vi "iTC_Readout (2).vi"() -> ()   [LabVIEW 2009]
panel:
  out "millisecond timer value":u32
  out "CCS Resistance":dynamicdata(graph)
  out "CCS Temperature":dbl(slide) scale=0.0..100.0
  in  "Samples Per Second 6":dbl=15.0
  out "CCS Temperature":string
  out "CCS Resistance":dbl(knob) scale=0.0..500.0
  out "CCS Resistance":string
  out "CCS Temperature":dynamicdata(graph)
  in  "Samples Per Second 5":dbl=15.0
  out "Allen Bradley Temperature":dbl(slide) scale=0.0..500.0
  out "Allen Bradley Temperature":string
  out "Allen Bradley Temperature":dynamicdata(graph)
  in  "Samples Per Second 4":dbl=15.0
  out "Allen Bradley Resistance":dbl(knob) scale=0.3..300.0
  out "Allen Bradley Resistance":string
  out "Allen Bradley Resistance":dynamicdata(graph)
  in  "Samples Per Second 3":dbl=15.0
  in  "Samples Per Second 2":dbl=15.0
  in  "Samples Per Second":dbl=15.0
  in  "stop 2":bool
  out "Heartbeat":bool
  out "Cernox Temp":string
  out "Cernox Temperature":dynamicdata(graph)
  out "Cernox Temp":dbl(slide) scale=0.0..320.0
  out "Cernox Resistance":dynamicdata(graph)
  out "Cernox Resistance":dbl(knob) scale=0.0..300.0
  out "Cernox Resistance":string
  in  "stop":bool
  out "Measurement":bool caption="Taken"
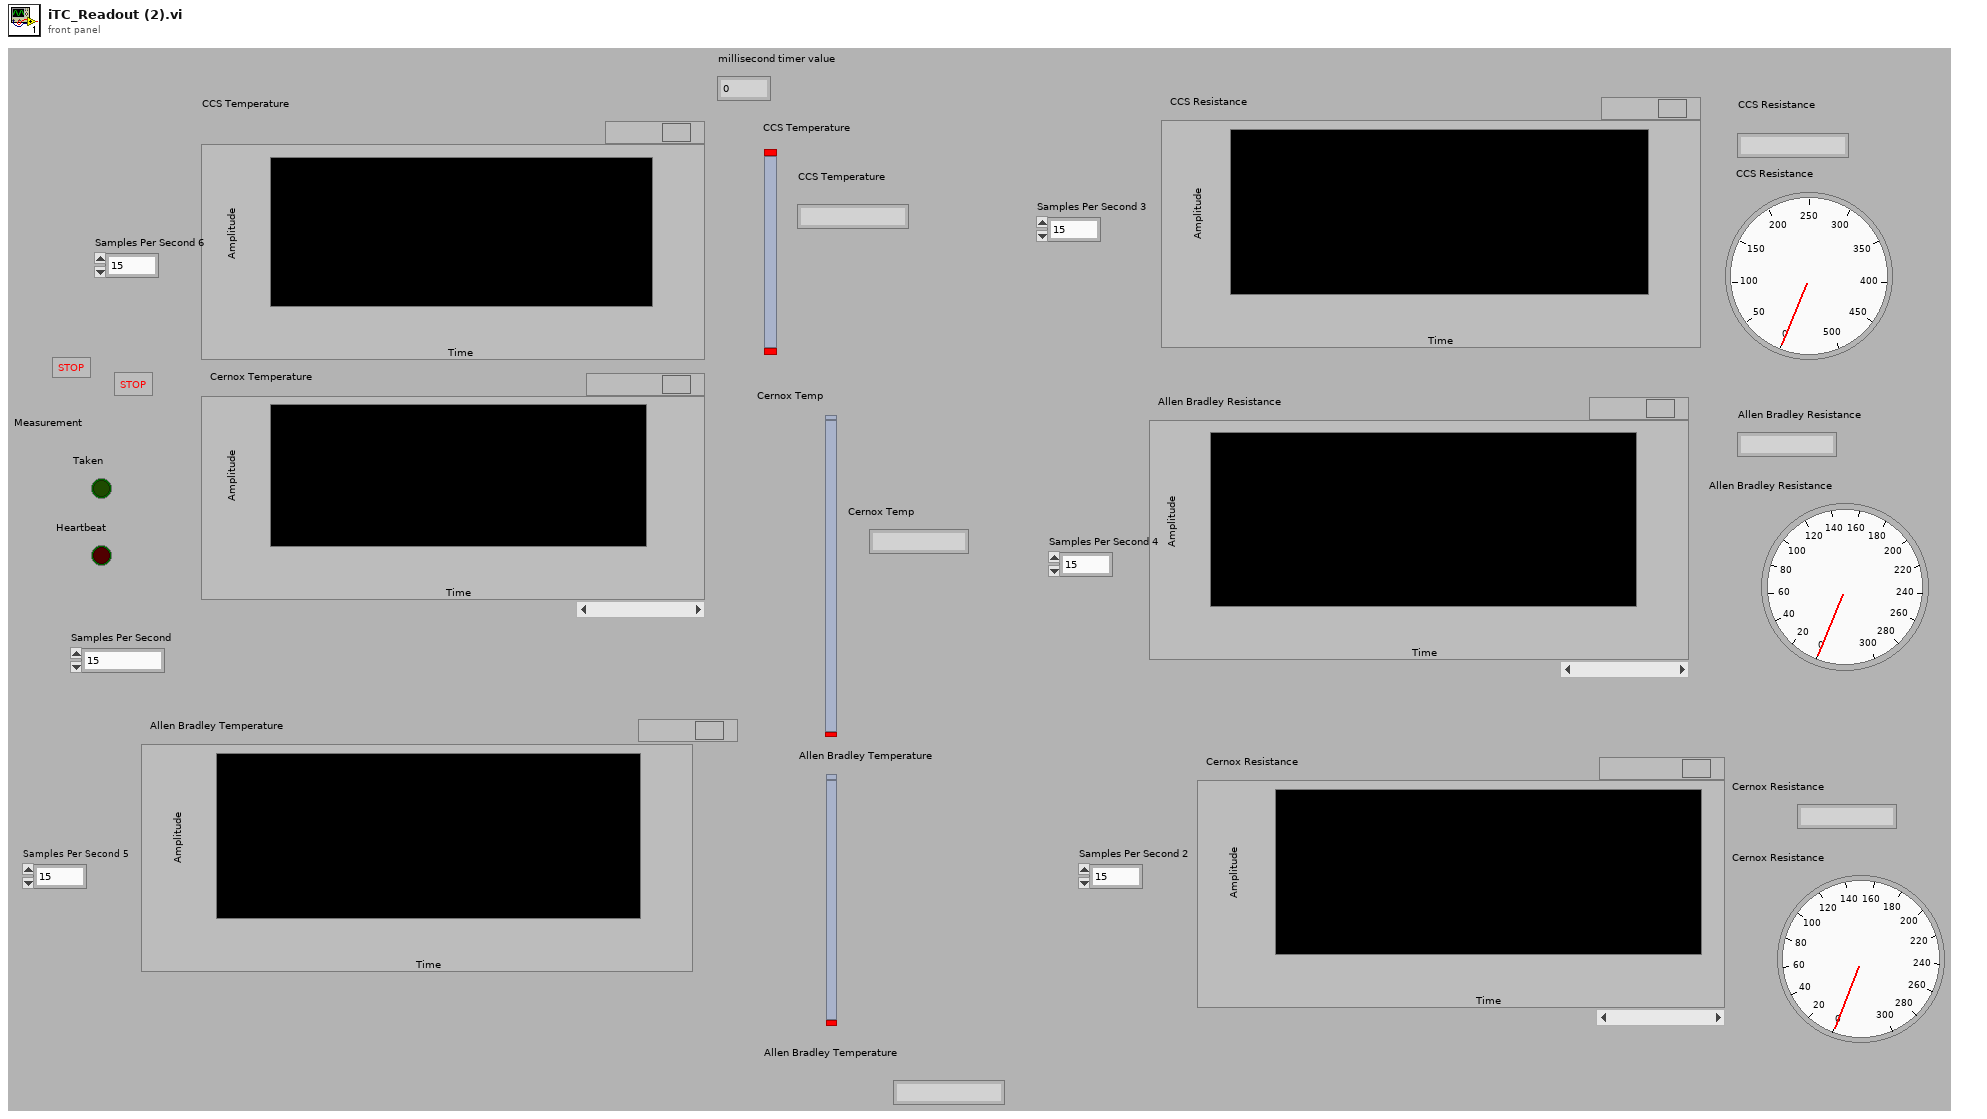
[diagram p1: front panel]
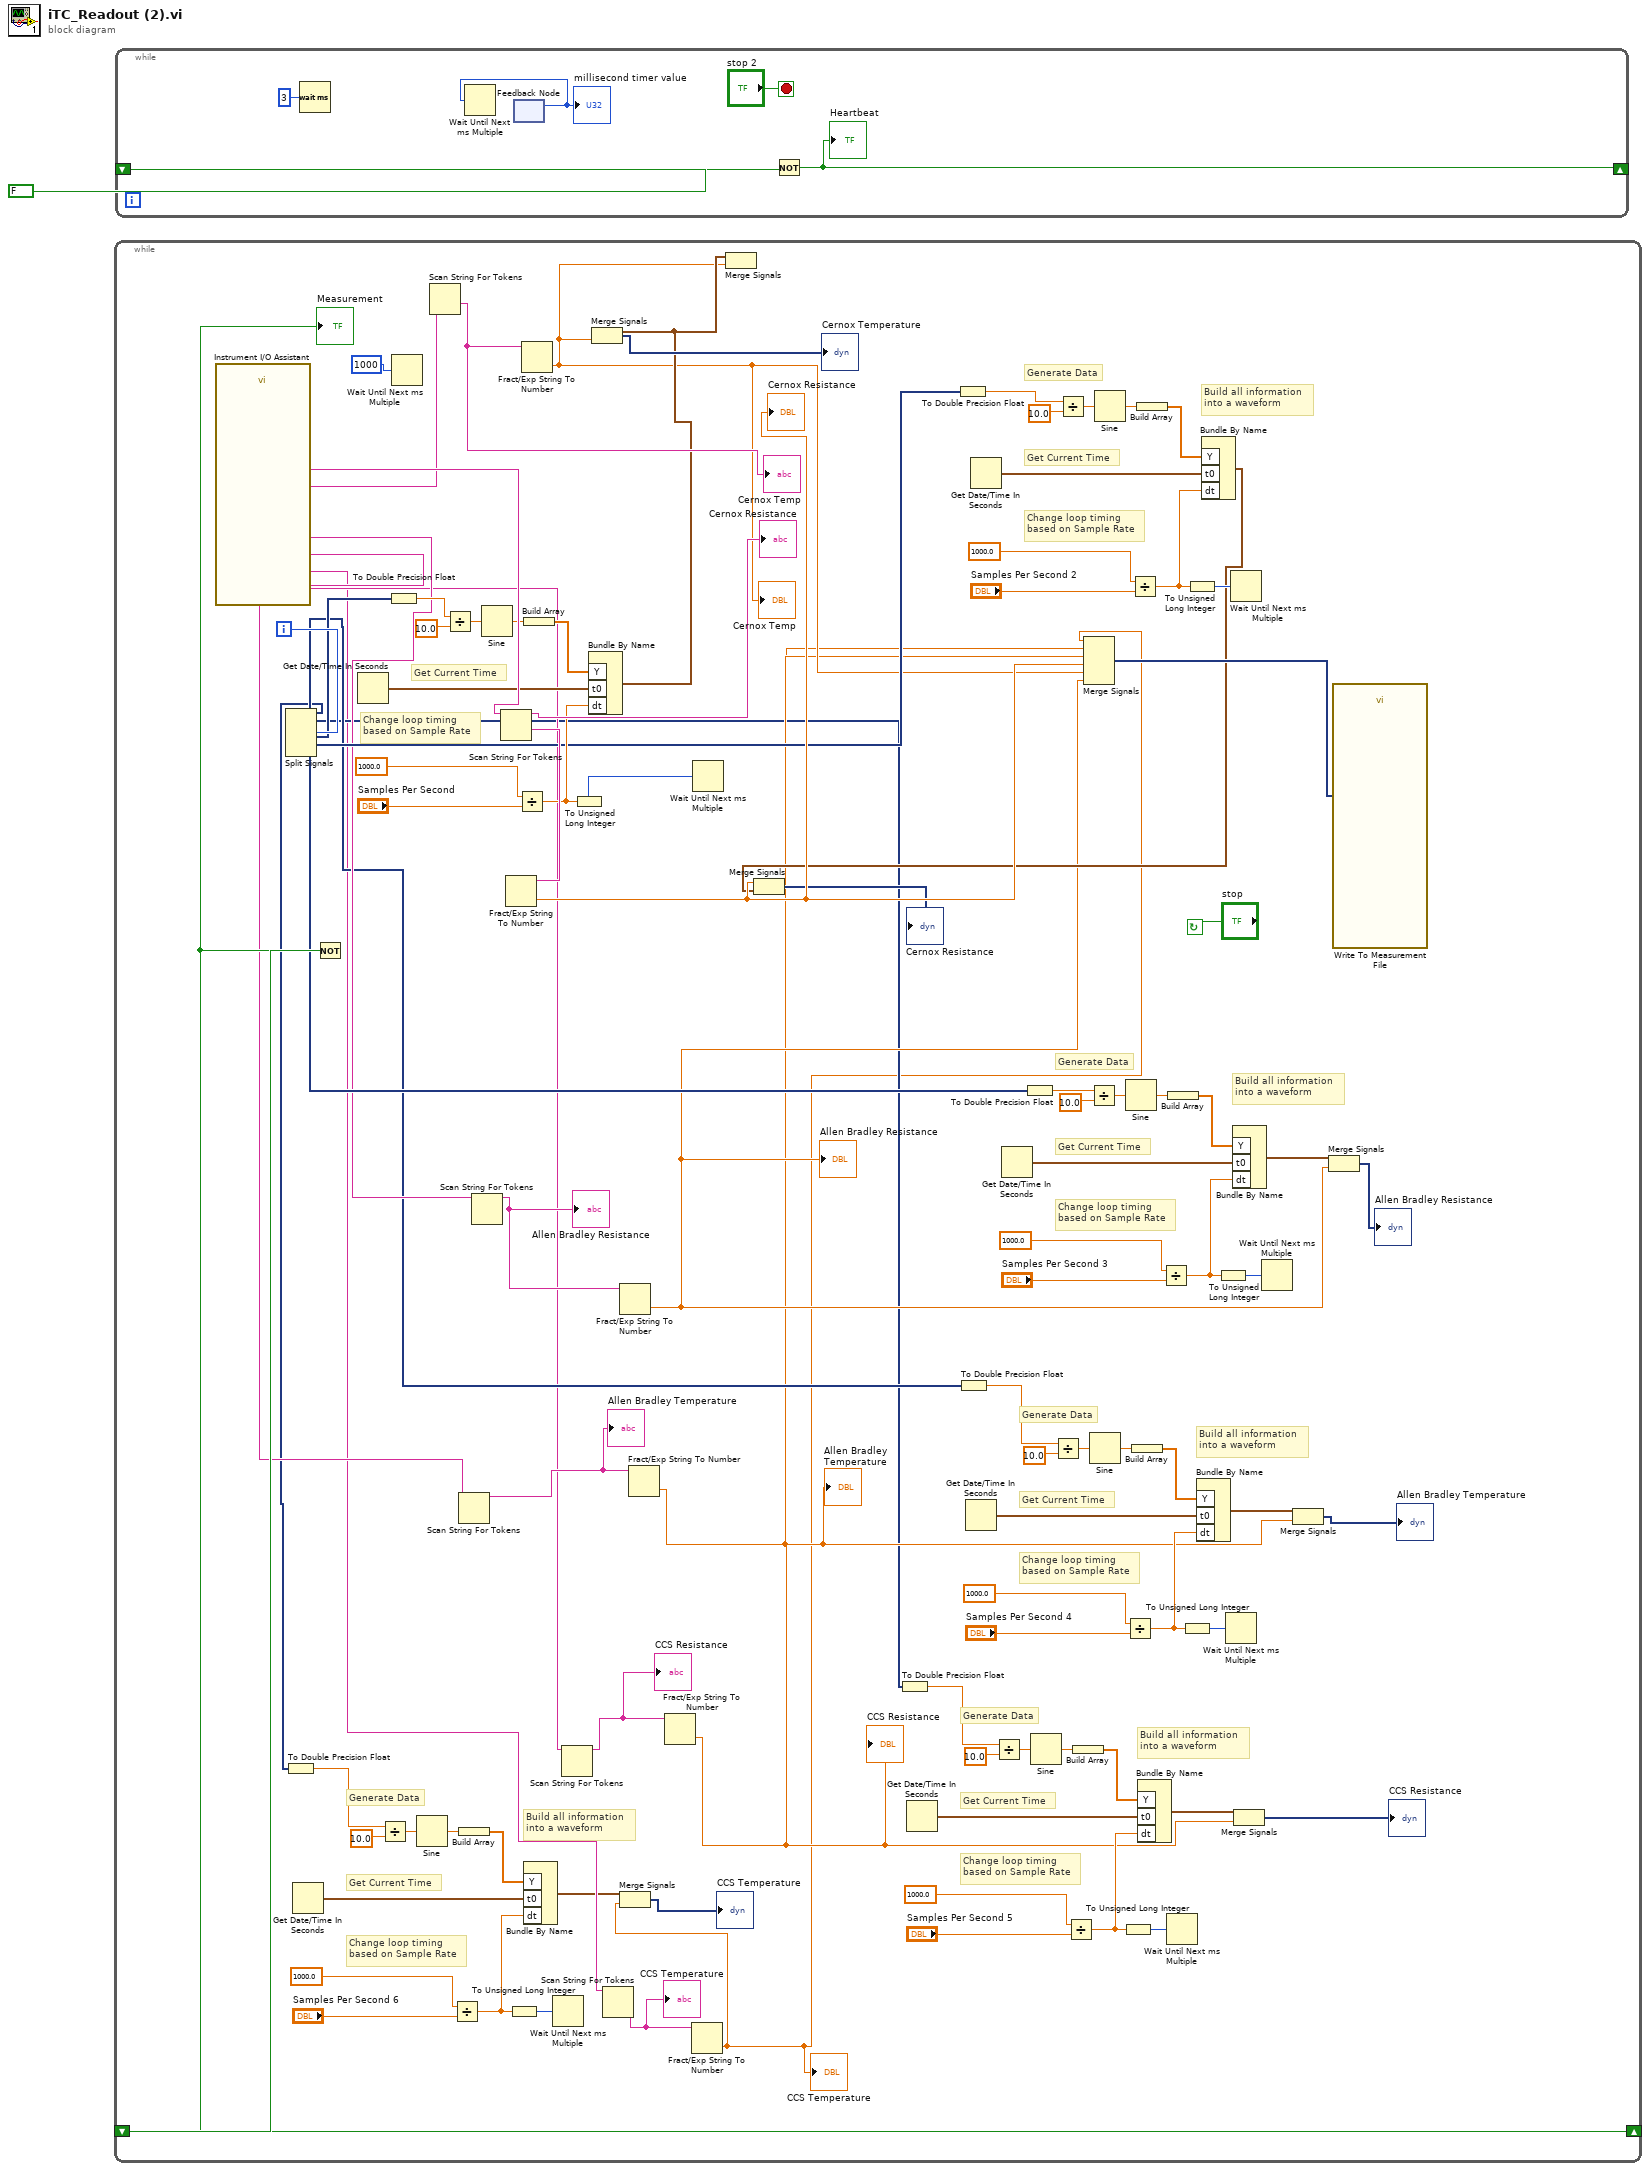
[diagram p0: block diagram]
diagram:
  n1 = while {
    shift-right: [w103] -> _
    shift-left: _ -> [w104]
    i -> [w70]
    stop <- "stop" continue-if-true
    # "Build all information\ninto a waveform"
    # "Change loop timing\nbased on Sample Rate"
    # "Get Current Time"
    # "Generate Data"
    # "Build all information\ninto a waveform"
    # "Change loop timing\nbased on Sample Rate"
    # "Get Current Time"
    # "Generate Data"
    # "Build all information\ninto a waveform"
    # "Change loop timing\nbased on Sample Rate"
    # "Get Current Time"
    # "Generate Data"
    # "Build all information\ninto a waveform"
    # "Change loop timing\nbased on Sample Rate"
    # "Get Current Time"
    # "Generate Data"
    # "Build all information\ninto a waveform"
    # "Change loop timing\nbased on Sample Rate"
    # "Get Current Time"
    # "Generate Data"
    # "Change loop timing\nbased on Sample Rate"
    # "Get Current Time"
    n2 = call "Instrument I/O Assistant"() -> ("token"=w22:string, "CCS Temperature"=w18:string, "Allen Bradley Temperature"=w37:string, "Allen Bradley Resistance"=w53:string, "Cernox Temp"=w99:string, "Cernox Resistance"=w101:string)  [unwired: 21 in, 1 out]
    n3 = Split Signals(w70) -> (w4:dynamicdata, w20:dynamicdata, w35:dynamicdata, w69:dynamicdata, w68:dynamicdata, w55:dynamicdata)  [unwired: 6 in]
    n4 = To Double Precision Float(number=w4) -> (double precision float=w10:dbl)
    n5 = Get Date/Time In Seconds() -> (seconds since 1Jan1904=w15:timestamp)
    n6 = Not(x=w104) -> (.not. x?=w103:bool)
    "Measurement" <- w103
    n7 = Get Date/Time In Seconds() -> (seconds since 1Jan1904=w85:timestamp)
    n8 = Divide(x=w10, y=10.0) -> (x/y=w7:dbl)
    n9 = To Double Precision Float(number=w69) -> (double precision float=w90:dbl)
    n10 = Wait Until Next ms Multiple(millisecond multiple=u32 1000) -> ()  [unwired: 1 out]
    n11 = Sine(x=w7) -> (sin(x)=w13:dbl)
    n12 = Scan String For Tokens(9:w99) -> (1:w97:string)  [unwired: 5 in, 3 out]
    "Cernox Temp" <- w97
    n13 = Divide(x=w90, y=10.0) -> (x/y=w93:dbl)
    n14 = Divide(x=1000.0, y="Samples Per Second 6") -> (x/y=w16:dbl)
    n15 = Scan String For Tokens(9:w37) -> (3:w36:string)  [unwired: 5 in, 3 out]
    "Allen Bradley Temperature" <- w36
    n16 = Build Array(w13) -> (w14:dbl[])
    n17 = Scan String For Tokens(9:w53) -> (3:w51:string)  [unwired: 5 in, 3 out]
    "Allen Bradley Resistance" <- w51
    n18 = Sine(x=w93) -> (sin(x)=w87:dbl)
    n19 = Scan String For Tokens(9:w101) -> (1:w100:string, 3:→"Cernox Resistance":string)  [unwired: 5 in, 2 out]
    n20 = Fract/Exp String To Number(string=w100) -> (number=w73:dbl)  [unwired: 3 in, 1 out]
    "Cernox Resistance" <- w73
    n21 = To Unsigned Long Integer(number=w16) -> (unsigned 32bit integer=w9:u32)
    n22 = Divide(x=1000.0, y="Samples Per Second") -> (x/y=w84:dbl)
    n23 = Fract/Exp String To Number(string=w97) -> (number=w66:dbl)  [unwired: 3 in, 1 out]
    "Cernox Temp" <- w66
    n24 = Build Array(w87) -> (w86:dbl[])
    n25 = Bundle By Name("Y"=w14, "t0"=w15, "dt"=w16) -> (w6:waveform(dbl))  [unwired: 1 in]
    n26 = Wait Until Next ms Multiple(millisecond multiple=w9) -> ()  [unwired: 1 out]
    n27 = Scan String For Tokens(9:w22) -> (3:w21:string)  [unwired: 5 in, 3 out]
    "CCS Resistance" <- w21
    n28 = To Unsigned Long Integer(number=w84) -> (unsigned 32bit integer=w91:u32)
    n29 = Bundle By Name("Y"=w86, "t0"=w85, "dt"=w84) -> (w67:waveform(dbl))  [unwired: 1 in]
    n30 = Merge Signals(w67, w66) -> (→"Cernox Temperature":dynamicdata)
    n31 = Scan String For Tokens(9:w18) -> (3:w17:string)  [unwired: 5 in, 3 out]
    "CCS Temperature" <- w17
    n32 = Fract/Exp String To Number(string=w51) -> (number=w50:dbl)  [unwired: 3 in, 1 out]
    "Allen Bradley Resistance" <- w50
    n33 = Fract/Exp String To Number(string=w36) -> (number=w34:dbl)  [unwired: 3 in, 1 out]
    "Allen Bradley Temperature" <- w34
    n34 = Fract/Exp String To Number(string=w21) -> (number=w19:dbl)  [unwired: 3 in, 1 out]
    "CCS Resistance" <- w19
    n35 = Fract/Exp String To Number(string=w17) -> (number=w3:dbl)  [unwired: 3 in, 1 out]
    "CCS Temperature" <- w3
    n36 = Merge Signals(w6, w3) -> (→"CCS Temperature":dynamicdata)
    n37 = Wait Until Next ms Multiple(millisecond multiple=w91) -> ()  [unwired: 1 out]
    n38 = Merge Signals(w67, w66) -> ()  [unwired: 1 out]
    n39 = To Double Precision Float(number=w20) -> (double precision float=w27:dbl)
    n40 = Get Date/Time In Seconds() -> (seconds since 1Jan1904=w32:timestamp)
    n41 = To Double Precision Float(number=w68) -> (double precision float=w77:dbl)
    n42 = To Double Precision Float(number=w35) -> (double precision float=w43:dbl)
    n43 = Get Date/Time In Seconds() -> (seconds since 1Jan1904=w48:timestamp)
    n44 = Get Date/Time In Seconds() -> (seconds since 1Jan1904=w82:timestamp)
    n45 = Divide(x=w27, y=10.0) -> (x/y=w24:dbl)
    n46 = Get Date/Time In Seconds() -> (seconds since 1Jan1904=w64:timestamp)
    n47 = To Double Precision Float(number=w55) -> (double precision float=w59:dbl)
    n48 = Sine(x=w24) -> (sin(x)=w30:dbl)
    n49 = Divide(x=w43, y=10.0) -> (x/y=w40:dbl)
    n50 = Divide(x=w77, y=10.0) -> (x/y=w74:dbl)
    n51 = Divide(x=1000.0, y="Samples Per Second 5") -> (x/y=w33:dbl)
    n52 = Build Array(w30) -> (w31:dbl[])
    n53 = Merge Signals(w3, w19, w34, w73, w66, w50) -> (w98:dynamicdata)
    n54 = Divide(x=w59, y=10.0) -> (x/y=w56:dbl)
    n55 = Sine(x=w40) -> (sin(x)=w46:dbl)
    n56 = Sine(x=w74) -> (sin(x)=w80:dbl)
    n57 = To Unsigned Long Integer(number=w33) -> (unsigned 32bit integer=w26:u32)
    n58 = Divide(x=1000.0, y="Samples Per Second 4") -> (x/y=w49:dbl)
    n59 = Sine(x=w56) -> (sin(x)=w62:dbl)
    n60 = Divide(x=1000.0, y="Samples Per Second 2") -> (x/y=w83:dbl)
    n61 = Build Array(w46) -> (w47:dbl[])
    n62 = Build Array(w80) -> (w81:dbl[])
    n63 = Bundle By Name("Y"=w31, "t0"=w32, "dt"=w33) -> (w23:waveform(dbl))  [unwired: 1 in]
    n64 = Divide(x=1000.0, y="Samples Per Second 3") -> (x/y=w65:dbl)
    n65 = Wait Until Next ms Multiple(millisecond multiple=w26) -> ()  [unwired: 1 out]
    n66 = Build Array(w62) -> (w63:dbl[])
    n67 = To Unsigned Long Integer(number=w49) -> (unsigned 32bit integer=w42:u32)
    n68 = To Unsigned Long Integer(number=w83) -> (unsigned 32bit integer=w76:u32)
    n69 = Bundle By Name("Y"=w47, "t0"=w48, "dt"=w49) -> (w39:waveform(dbl))  [unwired: 1 in]
    n70 = Bundle By Name("Y"=w81, "t0"=w82, "dt"=w83) -> (w71:waveform(dbl))  [unwired: 1 in]
    n71 = Merge Signals(w73, w71) -> (→"Cernox Resistance":dynamicdata)
    n72 = To Unsigned Long Integer(number=w65) -> (unsigned 32bit integer=w58:u32)
    n73 = Wait Until Next ms Multiple(millisecond multiple=w42) -> ()  [unwired: 1 out]
    n74 = Wait Until Next ms Multiple(millisecond multiple=w76) -> ()  [unwired: 1 out]
    n75 = Bundle By Name("Y"=w63, "t0"=w64, "dt"=w65) -> (w54:waveform(dbl))  [unwired: 1 in]
    n76 = Merge Signals(w23, w19) -> (→"CCS Resistance":dynamicdata)
    n77 = Wait Until Next ms Multiple(millisecond multiple=w58) -> ()  [unwired: 1 out]
    n78 = Merge Signals(w39, w34) -> (→"Allen Bradley Temperature":dynamicdata)
    n79 = Merge Signals(w54, w50) -> (→"Allen Bradley Resistance":dynamicdata)
    n80 = call "Write To Measurement File"("Signals"=w98) -> ()  [unwired: 16 in, 3 out]
  }
  n81 = while {
    shift-right: [w109] -> _
    shift-left: FALSE -> [w110]
    stop <- "stop 2" stop-if-true
    n82 = Wait (ms)(milliseconds to wait=u32 3) -> ()  [unwired: 1 out]
    n83 = feedback #1() -> (w106:u32)  [unwired: 1 in]
    "millisecond timer value" <- w106
    n84 = Wait Until Next ms Multiple(millisecond multiple=w106) -> (millisecond timer value=w107:u32)
    n85 = Not(x=w110) -> (.not. x?=w109:bool)
    "Heartbeat" <- w109
  }
